vi "z closure reply call.vi"(8 "error in (no error)":errorcluster, 10 "reply":cluster{}, 11 "closure":cluster{}) -> (0 "error out":errorcluster, 2 "reply out":cluster{})   [LabVIEW 2021, in "zenohc.lvlib"]
doc: "void z_closure_reply_call(const struct z_loaned_closure_reply_t *closure,\n struct z_loaned_reply_t *reply);"
uses:
  zenohc.lvlib
  zenohc.dll
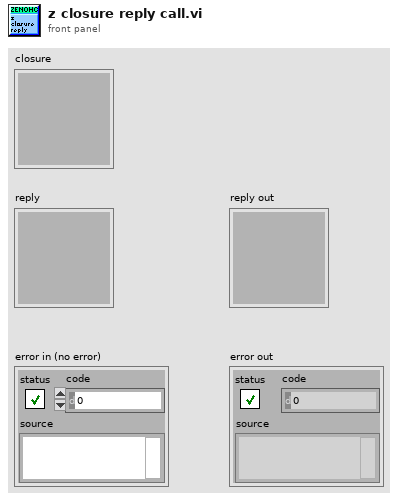
[diagram p1: front panel]
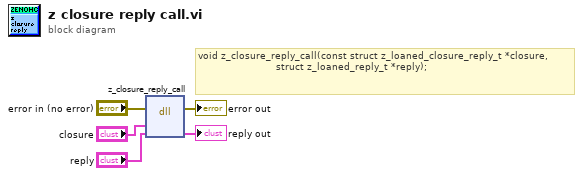
[diagram p0: block diagram]
diagram:
  # "void z_closure_reply_call(const struct z_loaned_closure_reply_t *closure,\n                          struct z_loaned_reply_t *reply);"
  n1 = dll-call lib="D:/dev/zenoh_labview/zenohc/zenohc.*" fn="z_closure_reply_call"(error in="error in (no error)", "closure"="closure", "reply"="reply") -> (error out=→"error out":errorcluster, "reply"=→"reply out":cluster{})  [unwired: 4 in, 1 out]
